vi "MAIN_CALLED_TESTASICS.vi"(8 "Error In":errorcluster, 11 "VISA resource name out":refnum<visa-resource-name>) -> (0 "Error Out":errorcluster)   [LabVIEW 2019]
uses:
  Type_defs/State_main.ctl
  LVPROJ_CONFIG_ESTACION/Type_defs/Coordenadas_estacion.ctl
  LVPROJ_CREAR BANDEJAS/Type_defs/Data_Bandeja.ctl
  Type_defs/INPUT TEST.ctl
  Type_defs/OUTPUTS_TEST.ctl
  LVPROJ_MOVIMIENTO_CABEZAL/LABVIEW_MOVIMIENTO/MOVIMIENTO CABEZAL/Typedefs/Comandos.ctl
  LVPROJ_MOVIMIENTO_CABEZAL/LABVIEW_MOVIMIENTO/MOVIMIENTO CABEZAL/Typedefs/Estados_arduino.ctl
  <vilib>/Utility/error.llb/Error Cluster From Error Code.vi
  <vilib>/ErrorRing/Error Ring.xnode
  SHARED VI'S/SHARED VI'S.lvlib
panel:
  out "trama datos enviada":string
  out "datos leídos por arduino":string
  in  "Tab Control":enum32{"PANEL USUARIO", "VER CONFIG ACTUAL"}(tab)
  in  "COMENZAR TEST":bool
  in  "EXIT":bool
  in  "DETENER TEST":bool
  in  "ENVIAR PARAMETROS DE TEST":bool
  in  "TEST ASICS INPUT":T1={"COORD. IN X"=0, "COORD IN Y"=0, "COORD OK X"=0, "COORD OK Y"=0, "COORD NOK X"=0, "COORD NOK Y"=0, "NºASICS A TESTEAR"=1, "SELECCIÓN DE TEST"=enum."TEST ASICS LST", "CUENTA ASICS"=0, "OPERADOR"="Javier Morales"}
  out "INDICADORES DE TEST":T2
  out "ESTADO FSM":T3
  in  "Path Out Reporte":path=path "C:/Trabajo_Robot/QC_LSTSUR"
  in  "Config file ASICS":path=path "C:/Trabajo_Robot/Test Asic Javi_2021/Origen Socket SERVO_PCB_BUENO_v5 (muchos asics)/CONFIG/configuracion_robot_CTAV2022A.test"
  in  "DIRECTORIO LOG FILE":path=path "C:/Trabajo_Robot/QC_LSTSUR/LOG/registro.txt"
  out "Configuracion Estación":T4={"Coordenadas_estacion"={"Coord.Bandeja entrada"={"Coord. X0 entrada"=0, "Coord. Y0 entrada "=0, "Altura Z entrada"=0}, "Coord.Bandeja OK"={"Coord. X0 OK"=0, "Coord. Y0 OK"=0, "Altura Z OK"=0}, "Coord.Bandeja entrada FAIL"={"Coord. X0 FAIL"=0, "Coord. Y0 FAIL"=0, "Altura Z FAIL"=0}, "Coord. Socket"={"Coord. X socket"=0, "Coord. Y socket"=0, "Altura Z socket"=0}}, "Nombre Bandeja"="", "Datos bandeja"={"Nº de columnas "=0, "Nº de filas "=0, "largo"=0, "ancho"=0, "nombre"="nombre", "Paso X (en mm)"=0.0, "Paso Y (en mm)"=0.0, "DISTANCIA SUELO A CHIP  "=0.0, "Nº de celdas totales"=0, "Distancia chips bandejas contiguas"=0.0}}
  out "read buffer":string
  out "read buffer 2":string
  out "datos enviados = datos leídos?":bool
  out "CONEXION CON ARDUINO":bool
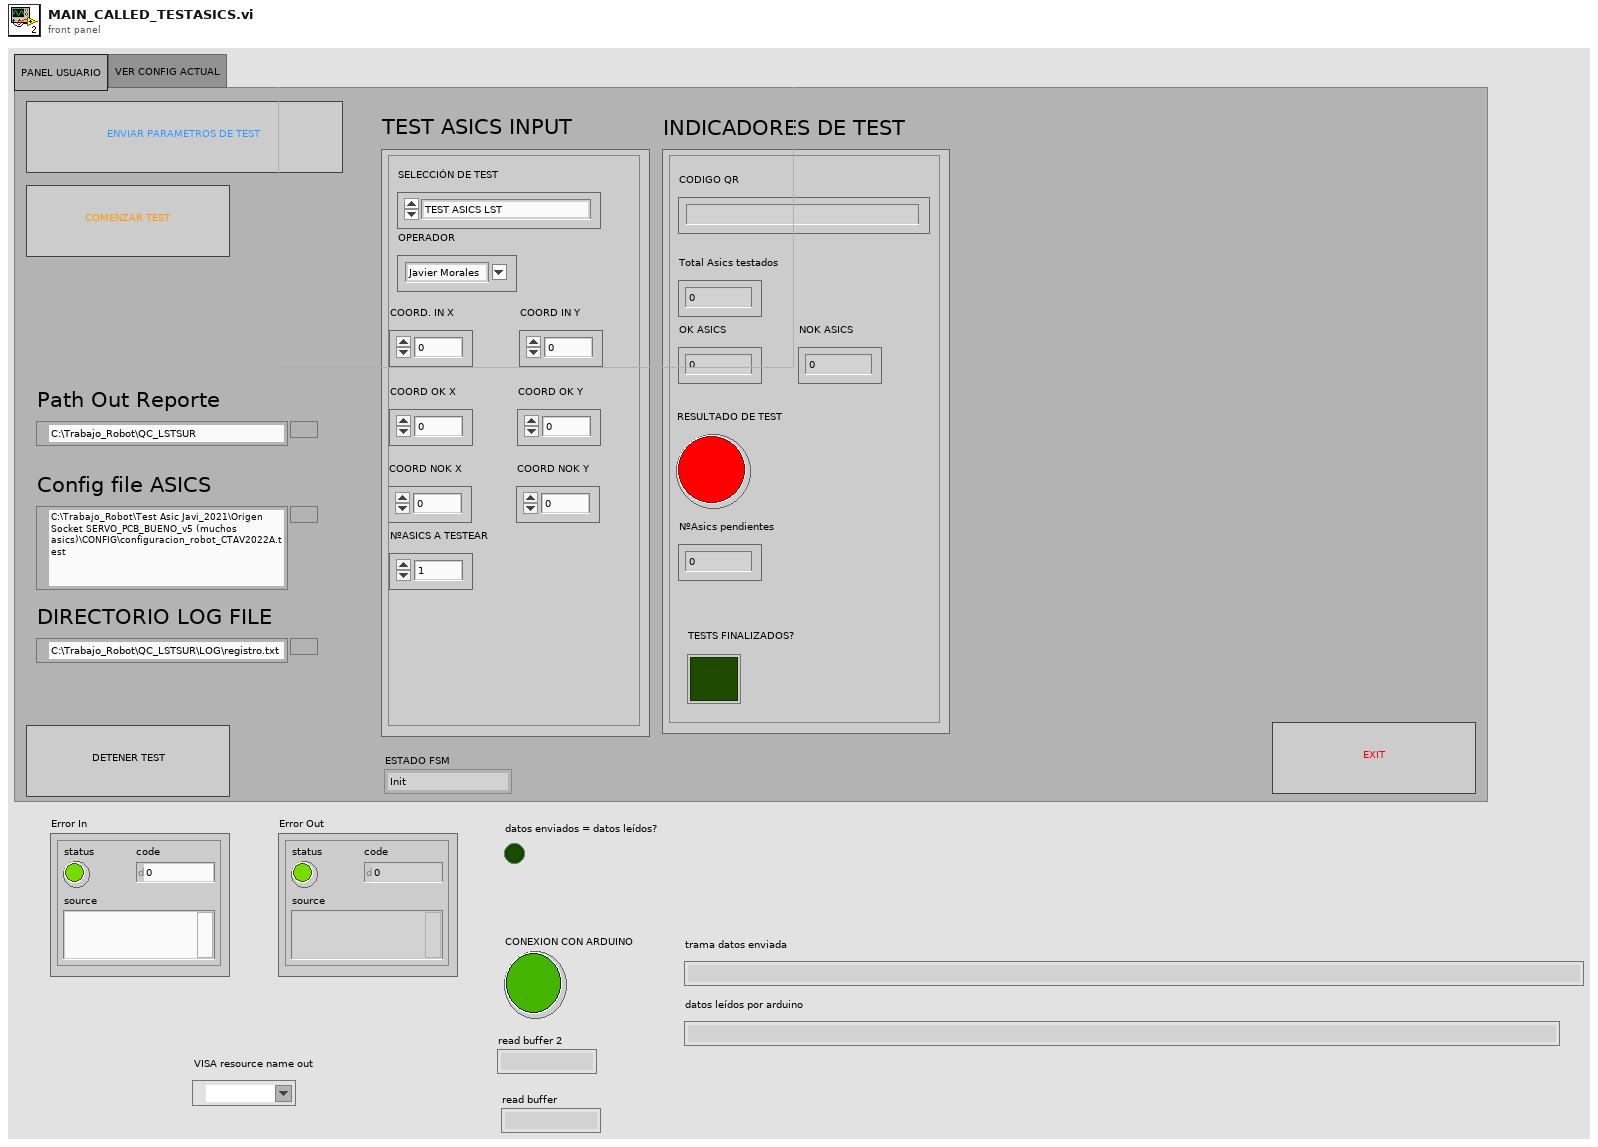
[diagram p1: front panel]
types:
  T1 = typedef "INPUT TEST.ctl" = cluster{"COORD. IN X":u16, "COORD IN Y":u16, "COORD OK X":u16, "COORD OK Y":u16, "COORD NOK X":u16, "COORD NOK Y":u16, "NºASICS A TESTEAR":u32, "SELECCIÓN DE TEST":enum16{"TEST ASICS LST"}, "CUENTA ASICS":u32, "OPERADOR":string}
  T2 = typedef "OUTPUTS_TEST.ctl" = cluster{"CODIGO QR":string, "OK ASICS":u32, "NOK ASICS":u32, "RESULTADO DE TEST":bool, "TESTS FINALIZADOS?":bool, "Total Asics testados":u32, "NºAsics pendientes":u32}
  T3 = typedef "State_main.ctl" = enum16{"Init", "Wait for Event", "Init refs", "Init com", "Config estacion", "Home", "Ping_Arduino", "Coge Asic", "Enviar_config_test", "Test_call", "Dejar Asic", "Leer QR", "Ejecutar Test", "Actualizar valores", "Enviar resultadoTest Arduino", "Final de test?", "Terminar", "Exit", "Error?"}
  T4 = typedef "Configuracion_estación.ctl" = cluster{"Coordenadas_estacion":T5, "Nombre Bandeja":string, "Datos bandeja":T6}
  T5 = typedef "Coordenadas_estacion.ctl" = cluster{"Coord.Bandeja entrada":cluster{"Coord. X0 entrada":u32, "Coord. Y0 entrada ":u32, "Altura Z entrada":u32}, "Coord.Bandeja OK":cluster{"Coord. X0 OK":u32, "Coord. Y0 OK":u32, "Altura Z OK":u32}, "Coord.Bandeja entrada FAIL":cluster{"Coord. X0 FAIL":u32, "Coord. Y0 FAIL":u32, "Altura Z FAIL":u32}, "Coord. Socket":cluster{"Coord. X socket":u32, "Coord. Y socket":u32, "Altura Z socket":u32}}
  T6 = typedef "Data_Bandeja.ctl" = cluster{"Nº de columnas ":u32, "Nº de filas ":u32, "largo":u32, "ancho":u32, "nombre":string, "Paso X (en mm)":dbl, "Paso Y (en mm)":dbl, "DISTANCIA SUELO A CHIP  ":dbl, "Nº de celdas totales":u16, "Distancia chips bandejas contiguas":dbl}
  T7 = typedef "Comandos.ctl" = enum16{"H", "FH", "FM", "FI", "FX", "FY", "FZ", "I", "OK"}
  T8 = typedef "Estados_arduino.ctl" = enum16{"2", "3", "4", "5", "6", "7", "9", "8"}
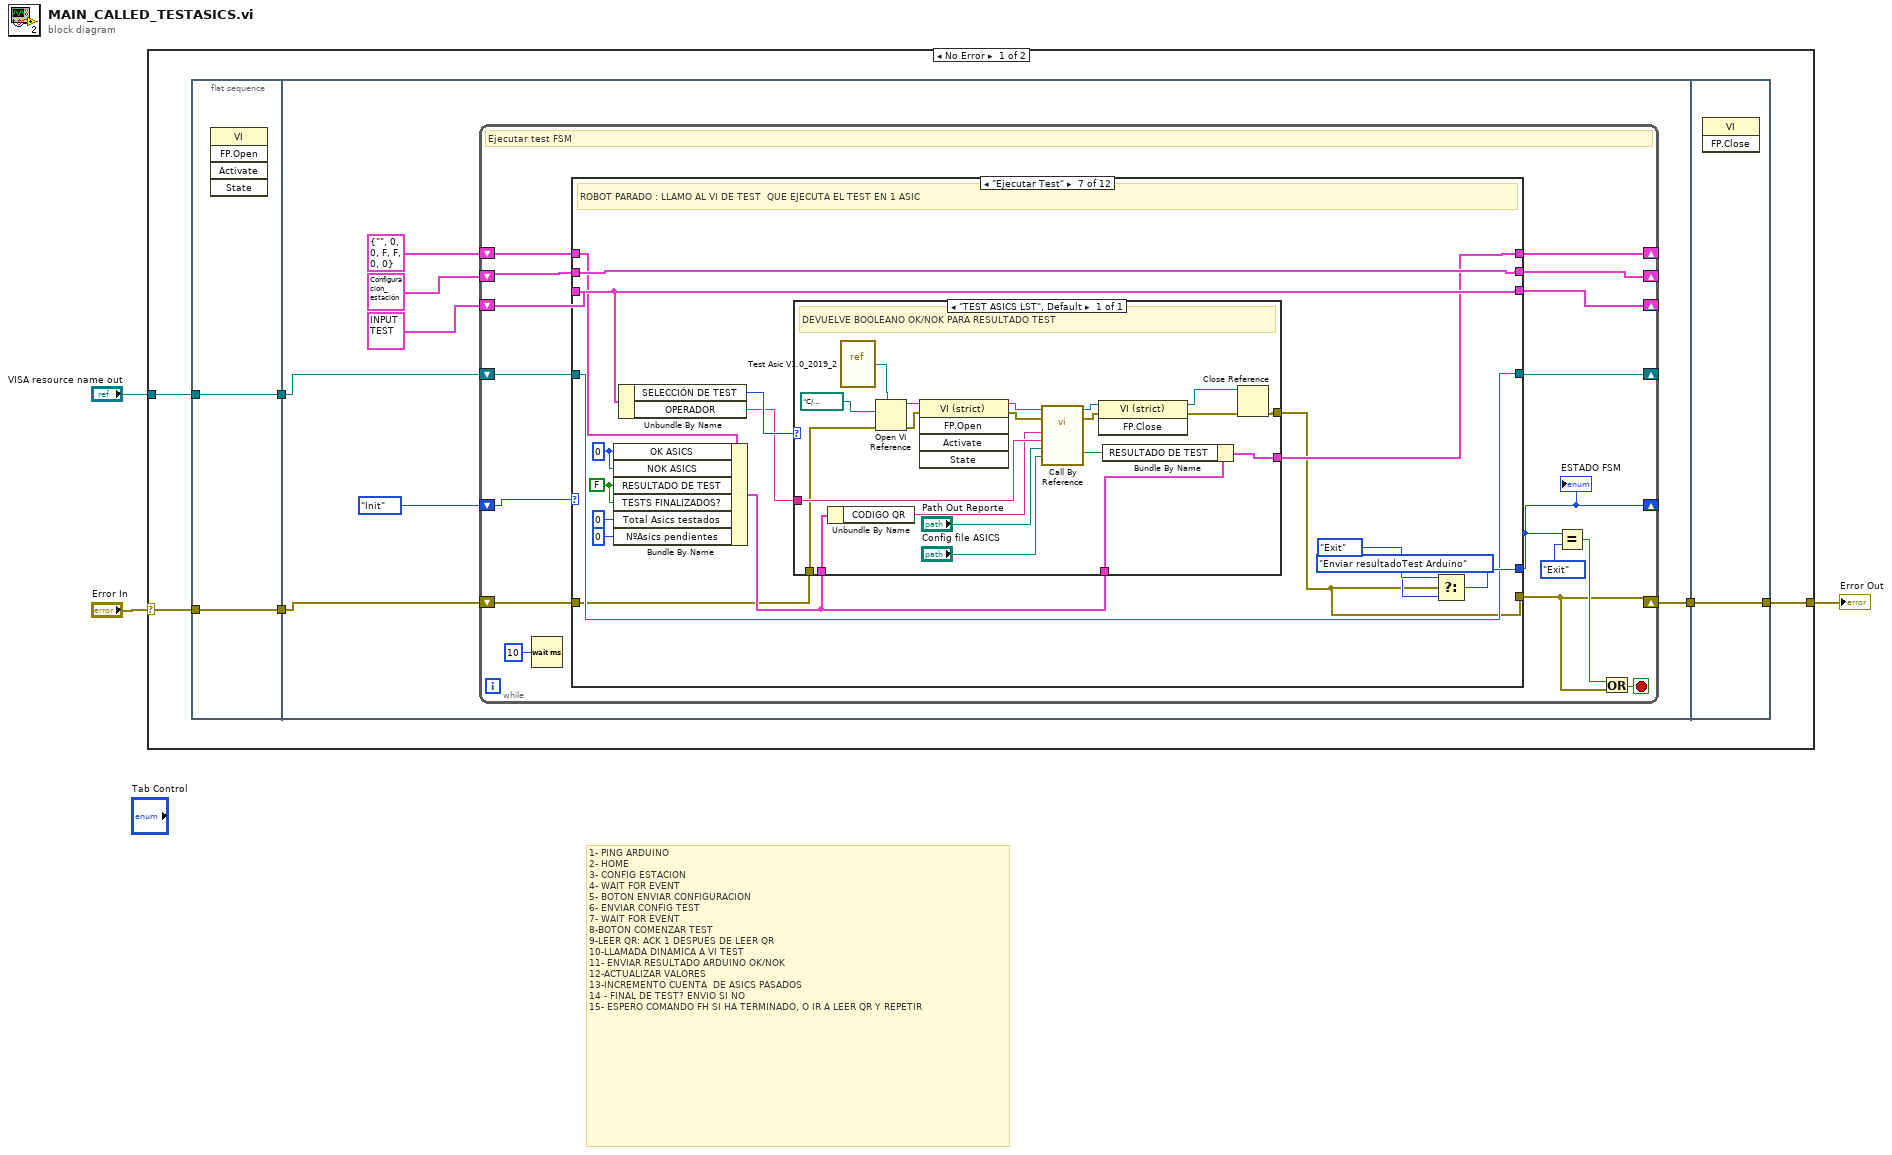
[diagram p0: block diagram]
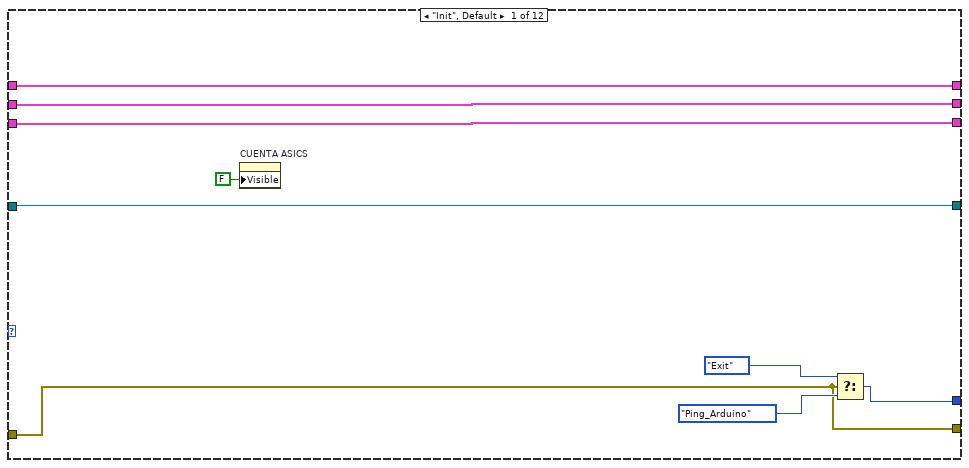
[diagram p2: hidden frame]
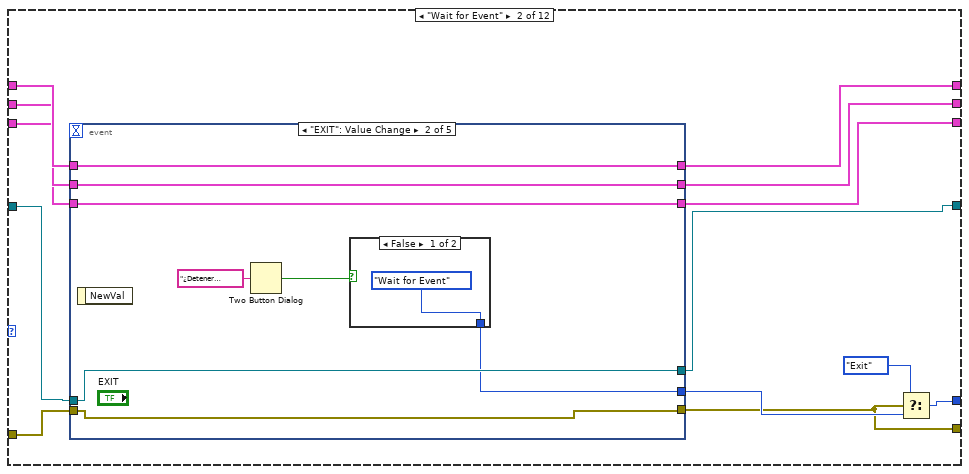
[diagram p3: hidden frame]
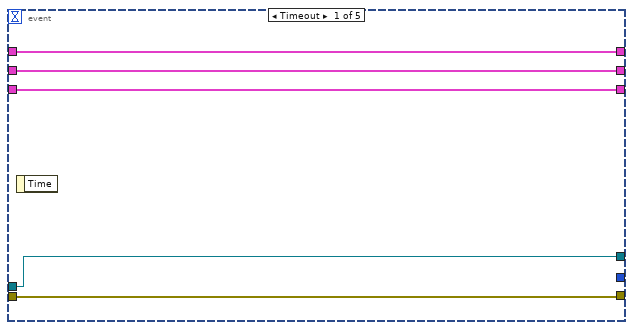
[diagram p4: hidden frame]
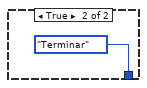
[diagram p5: hidden frame]
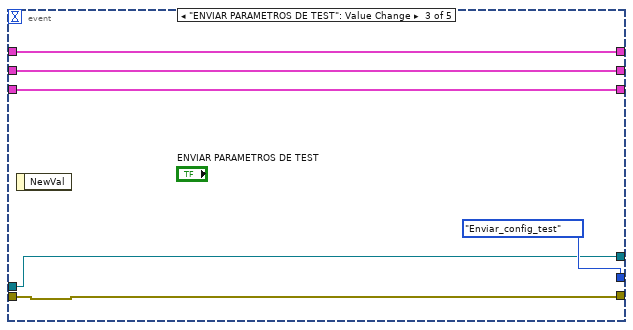
[diagram p6: hidden frame]
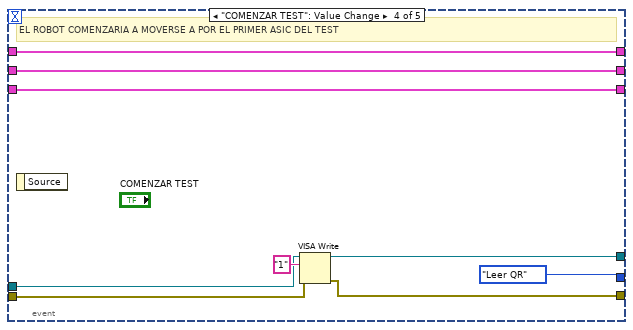
[diagram p7: hidden frame]
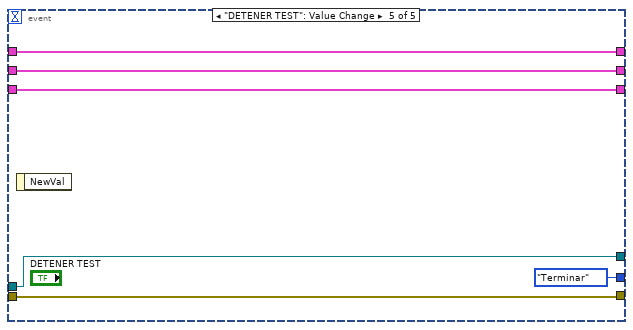
[diagram p8: hidden frame]
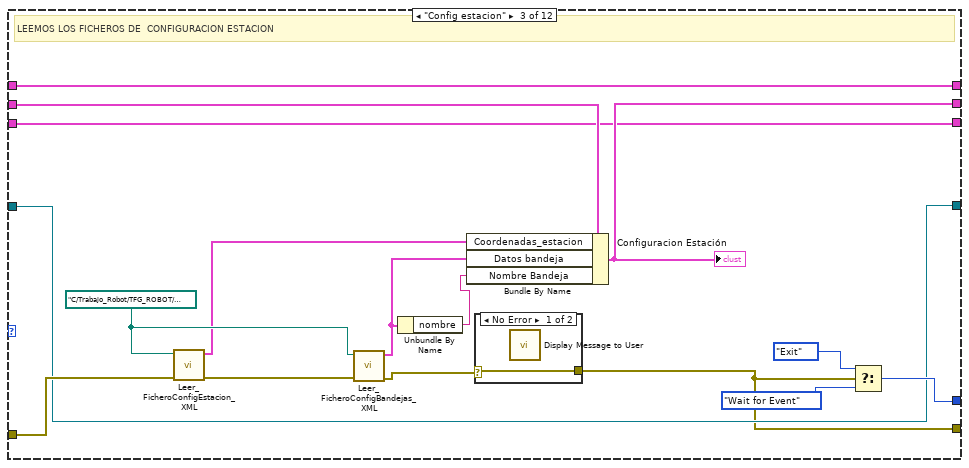
[diagram p9: hidden frame]
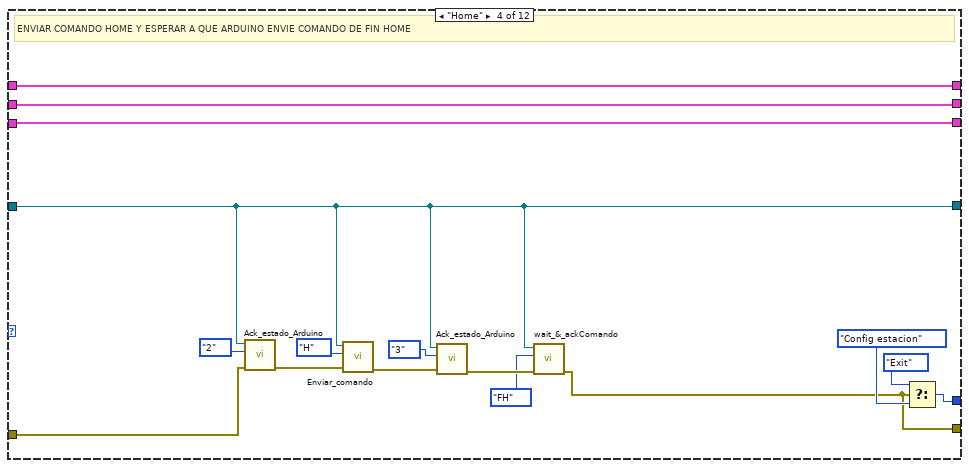
[diagram p11: hidden frame]
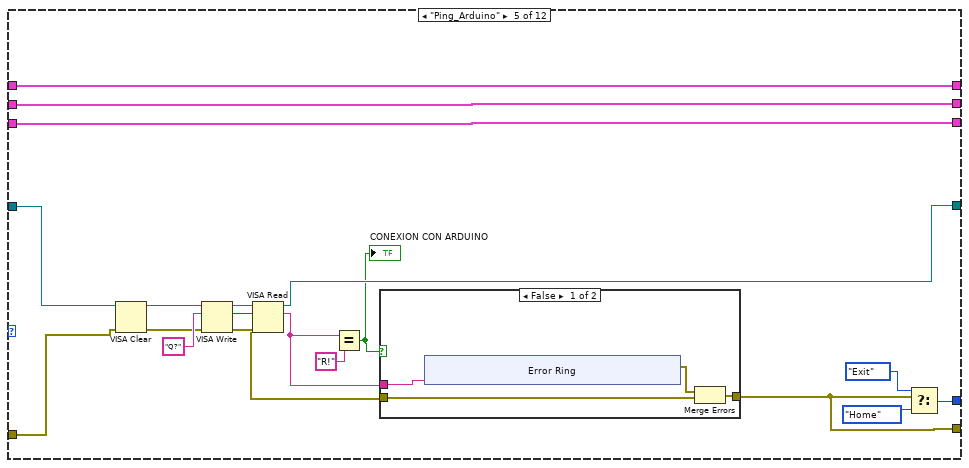
[diagram p12: hidden frame]
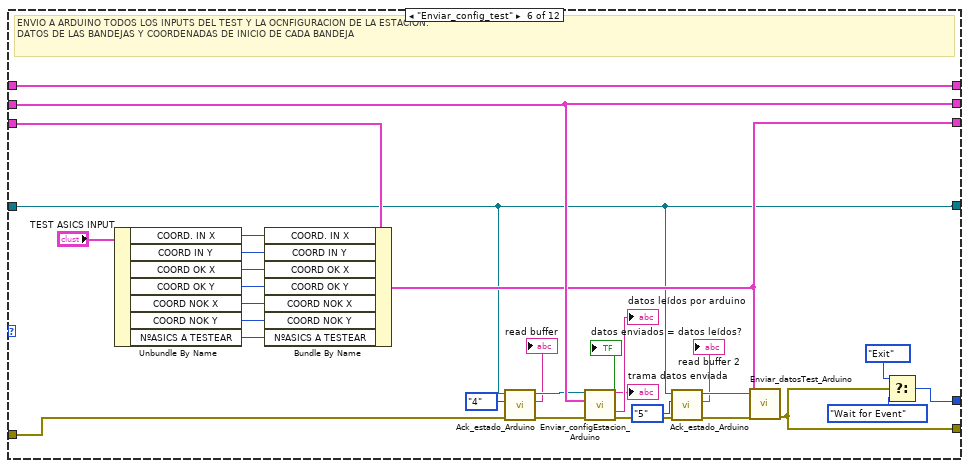
[diagram p14: hidden frame]
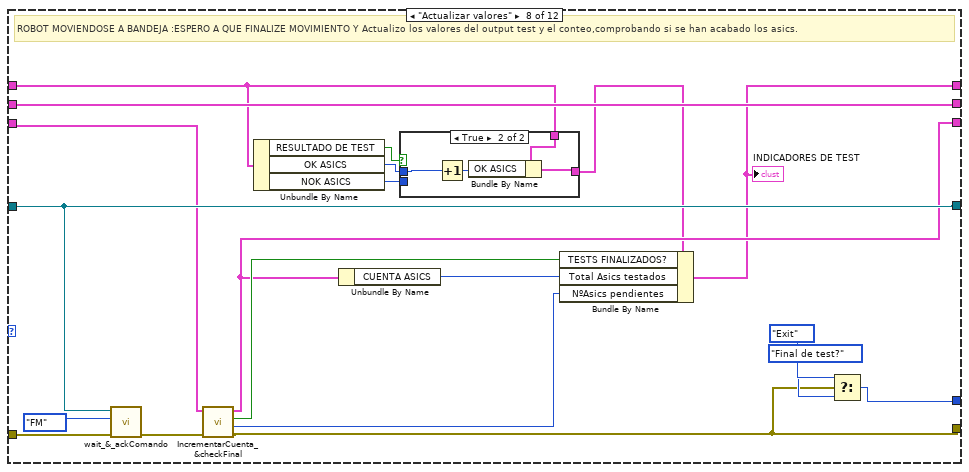
[diagram p15: hidden frame]
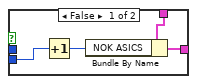
[diagram p16: hidden frame]
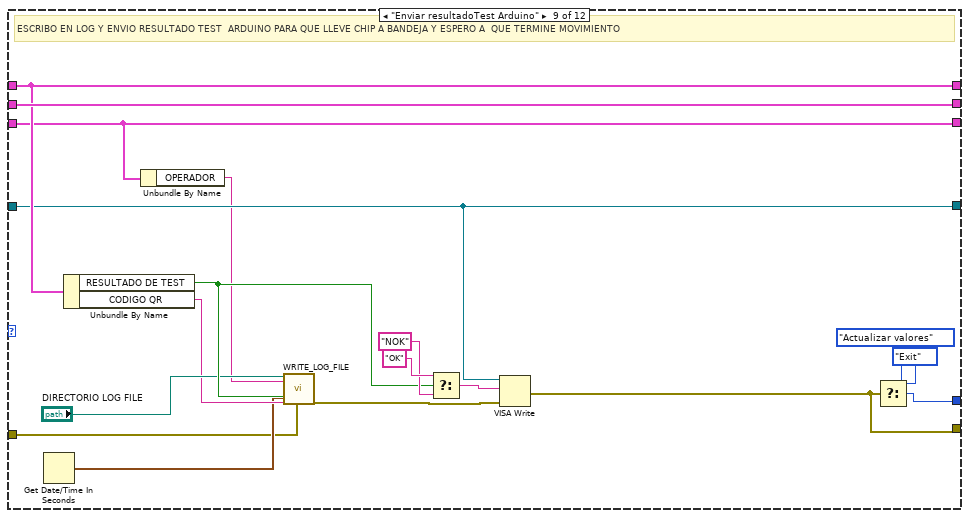
[diagram p17: hidden frame]
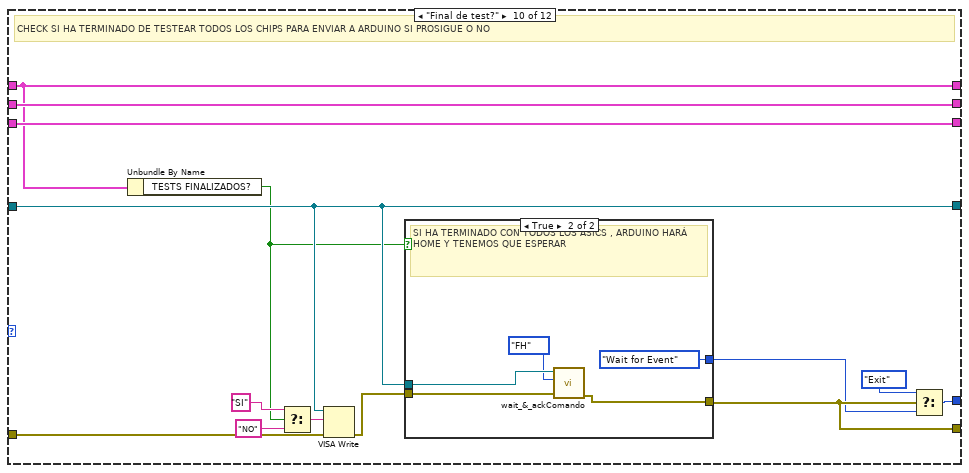
[diagram p18: hidden frame]
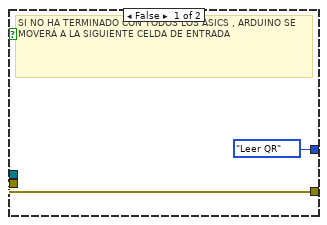
[diagram p19: hidden frame]
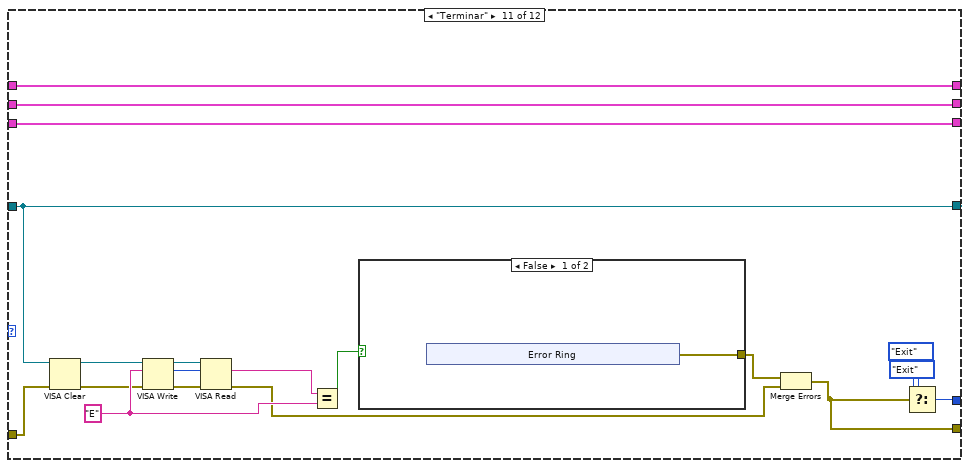
[diagram p20: hidden frame]
diagram:
  # "1- PING ARDUINO\n2- HOME\n3- CONFIG ESTACION\n4- WAIT FOR EVENT\n5- BOTON ENVIAR CONFIGURACION\n6- ENVIAR CONFIG TEST\n7- WAIT FOR EVENT\n8-BOTON COMENZAR TEST\n9-LEER QR: ACK 1 DESPUES DE LEER QR\n10-LLAMADA DINAMICA A VI TEST\n11- ENVIAR RESULTADO ARDUINO OK/NOK\n12-ACTUALIZAR VALORES\n13-INCREMENTO CUENTA  DE ASICS PASADOS\n14 - FINAL DE TEST? ENVIO SI NO\n15- ESPERO COMANDO FH SI HA TERMINADO, O IR A LEER QR Y REPETIR"
  n1 = case shown="No Error" "Error In" {
    selector: "Error In" -> [w9 w339]
    tunnel: "VISA resource name out" -> [w7 _]
    tunnel: [w4 w339] -> w1
    frame No Error {
      n2 = flat-sequence {
        tunnel: w9 -> [w11]
        tunnel: [w11] -> w8
        tunnel: w7 -> [w10]
        tunnel: [w10] -> w6
        tunnel: w8 -> [w14]
        tunnel: w6 -> [w13]
        tunnel: [w12] -> w5
        tunnel: w5 -> [w338]
        tunnel: [w338] -> w4
        frame #0 {
          n3 = invoke class="VI" method="FP.Open"() -> ()  [unwired: 5 in, 5 out]
        }
        frame #1 {
          n4 = while {
            shift-right: [w27] -> _
            shift-left: State_main."Init" ("States_main") -> [w34]
            shift-right: [w28] -> w12
            shift-left: w14 -> [w32]
            shift-right: [w20] -> _
            shift-left: T1 {"COORD. IN X"=0, "COORD IN Y"=0, "COORD OK X"=0, "COORD OK Y"=0, "COORD NOK X"=0, "COORD NOK Y"=0, "NºASICS A TESTEAR"=1, "SELECCIÓN DE TEST"=enum."TEST ASICS LST", "CUENTA ASICS"=0, "OPERADOR"="Javier Morales"} ("TEST ASICS INPUT") -> [w31]
            shift-right: [w22] -> _
            shift-left: T4 {"Coordenadas_estacion"={"Coord.Bandeja entrada"={"Coord. X0 entrada"=0, "Coord. Y0 entrada "=0, "Altura Z entrada"=0}, "Coord.Bandeja OK"={"Coord. X0 OK"=0, "Coord. Y0 OK"=0, "Altura Z OK"=0}, "Coord.Bandeja entrada FAIL"={"Coord. X0 FAIL"=0, "Coord. Y0 FAIL"=0, "Altura Z FAIL"=0}, "Coord. Socket"={"Coord. X socket"=0, "Coord. Y socket"=0, "Altura Z socket"=0}}, "Nombre Bandeja"="", "Datos bandeja"={"Nº de columnas "=0, "Nº de filas "=0, "largo"=0, "ancho"=0, "nombre"="nombre", "Paso X (en mm)"=0.0, "Paso Y (en mm)"=0.0, "DISTANCIA SUELO A CHIP  "=0.0, "Nº de celdas totales"=0, "Distancia chips bandejas contiguas"=0.0}} ("Configuracion Estación") -> [w26]
            shift-right: [w24] -> _
            shift-left: w13 -> [w25]
            shift-right: [w21] -> _
            shift-left: T2 {"CODIGO QR"="", "OK ASICS"=0, "NOK ASICS"=0, "RESULTADO DE TEST"=FALSE, "TESTS FINALIZADOS?"=FALSE, "Total Asics testados"=0, "NºAsics pendientes"=0} -> [w23]
            stop <- w30 stop-if-true
            # "Ejecutar test FSM"
            n5 = Wait (ms)(milliseconds to wait=u32 10) -> ()  [unwired: 1 out]
            n6 = case shown="\"Ejecutar Test\"" w34 {
              tunnel: w32 -> [w36 w47 w105 w114 w130 w171 w190 w240 w255 w278 w297 w328]
              tunnel: w31 -> [w38 w49 w95 w121 w141 w185 w200 w238 w258 w282 w307 w330]
              tunnel: [w41 w55 w106 w124 w144 w186 w203 w243 w269 w284 w306 w332] -> w27
              tunnel: [w36 w46 w93 w113 w133 w174 w189 w236 w262 w276 w293 w323] -> w28
              tunnel: w26 -> [w39 w51 w98 w122 w142 w175 w201 w242 w268 w283 w308 w331]
              tunnel: w25 -> [w37 w45 w99 w111 w128 w166 w199 w241 w263 w275 w296 w327]
              tunnel: [w37 w44 w99 w111 w132 w166 w199 w241 w263 w275 w296 w327] -> w24
              tunnel: w23 -> [w40 w53 w96 w123 w143 w176 w194 w229 w267 w272 w309 w326]
              tunnel: [w39 w50 w97 w122 w142 w175 w201 w242 w268 w283 w308 w331] -> w22
              tunnel: [w40 w52 w96 w123 w143 w176 w191 w231 w267 w272 w309 w325] -> w21
              tunnel: [w38 w48 w95 w121 w141 w173 w200 w234 w258 w282 w307 w330] -> w20
              frame "Init", Default {
                n7 = property on="CUENTA ASICS" class="DigNum (strict)"("Visible"=FALSE) -> ()  [unwired: 2 in, 2 out]
                n8 = Select(t=State_main."Exit" ("States_main"), s=w36, f=State_main."Ping_Arduino" ("States_main")) -> (s? t:f=w41:T3)
              }
              frame "Wait for Event" {
                n9 = event shown="[1] \"EXIT\": Value Change" {
                  selector: _ -> [_ _ _ _ _]
                  dyn-events: _ -> [_ _ _ _ _]
                  timeout: _ -> [_ _ _ _ _]
                  tunnel: [_ w62 State_main."Enviar_config_test" ("States_main") State_main."Leer QR" ("States_main") State_main."Terminar" ("States_main")] -> w54
                  tunnel: w53 -> [w61 w69 w76 w85 w92]
                  tunnel: [w61 w69 w76 w85 w92] -> w52
                  tunnel: w51 -> [w60 w68 w75 w84 w91]
                  tunnel: [w60 w68 w75 w84 w91] -> w50
                  tunnel: w49 -> [w59 w67 w74 w83 w90]
                  tunnel: [w59 w67 w74 w83 w90] -> w48
                  tunnel: w47 -> [w58 w66 w73 w79 w88]
                  tunnel: [w58 w66 w73 w78 w88] -> w46
                  tunnel: w45 -> [w57 w65 w72 w81 w87]
                  tunnel: [w57 w65 w72 w80 w87] -> w44
                  event Timeout {
                    n10 = event-data() -> ()  [unwired: 1 in, 1 out]
                  }
                  event "EXIT": Value Change {
                    n11 = event-data() -> ()  [unwired: 1 in, 1 out]
                    n12 = Two Button Dialog(message="¿Detener ejecución?") -> (T button?=w63:bool)  [unwired: 2 in]
                    n13 = case shown="False" w63 {
                      tunnel: [State_main."Wait for Event" ("States_main") State_main."Terminar" ("States_main")] -> w62
                      frame False {
                      }
                      frame True {
                      }
                    }
                  }
                  event "ENVIAR PARAMETROS DE TEST": Value Change {
                    n14 = event-data() -> ()  [unwired: 1 in, 1 out]
                  }
                  event "COMENZAR TEST": Value Change {
                    # "EL ROBOT COMENZARIA A MOVERSE A POR EL PRIMER ASIC DEL TEST"
                    n15 = event-data() -> ()  [unwired: 1 in, 1 out]
                    n16 = VISA Write(VISA resource name=w81, write buffer="1", error in (no error)=w79) -> (VISA resource name out=w80:refnum<visa-resource-name>, error out=w78:errorcluster)  [unwired: 1 out]
                  }
                  event "DETENER TEST": Value Change {
                    n17 = event-data() -> ()  [unwired: 1 in, 1 out]
                  }
                }
                n18 = Select(t=State_main."Exit" ("States_main"), s=w46, f=w54) -> (s? t:f=w55:T3)
              }
              frame "Config estacion" {
                w103 = path "C:/Trabajo_Robot/TFG_ROBOT/CONTROL_ROBOT/LABVIEW_ROBOT_MASTER" ("XML File Path")
                # "LEEMOS LOS FICHEROS DE  CONFIGURACION ESTACION"
                n19 = call "Leer_FicheroConfigEstacion_XML.vi"("error in (no error)"=w105, "XML File Path"=w103) -> ("error out"=w104:errorcluster, "Coordenadas_estacion"=w102:T5)  [unwired: 8 in]
                n20 = call "Leer_FicheroConfigBandejas_XML.vi"("error in (no error)"=w104, "XML File Path"=w103) -> ("error out"=w94:errorcluster, "Datos bandeja"=w101:T6)  [unwired: 8 in]
                n21 = Unbundle By Name(w101) -> ("nombre"=w100:string)
                n22 = Bundle By Name(cluster=w98, "Coordenadas_estacion"=w102, "Datos bandeja"=w101, "Nombre Bandeja"=w100) -> (w97:T4)
                "Configuracion Estación" <- w97
                n23 = case shown="No Error" w94 {
                  selector: w94 -> [w109 w110]
                  tunnel: [w109 w110] -> w93
                  frame No Error {
                    n24 = call "Display Message to User"() -> ()  [unwired: 10 in, 2 out]
                  }
                  frame Error {
                  }
                }
                n25 = Select(t=State_main."Exit" ("States_main"), s=w93, f=State_main."Wait for Event" ("States_main")) -> (s? t:f=w106:T3)
              }
              frame "Home" {
                # "ENVIAR COMANDO HOME Y ESPERAR A QUE ARDUINO ENVIE COMANDO DE FIN HOME"
                n26 = call "Ack_estado_Arduino.vi"("error in (no error)"=w114, "Enum"=Estados_arduino."2", "VISA resource name"=w111) -> ("error out"=w120:errorcluster)  [unwired: 6 in, 2 out]
                n27 = call "Enviar_comando.vi"("error in (no error)"=w120, "Enum"=Comandos."H", "VISA resource name"=w111) -> ("error out"=w115:errorcluster)  [unwired: 6 in, 2 out]
                n28 = call "Ack_estado_Arduino.vi"("error in (no error)"=w115, "Enum"=Estados_arduino."3", "VISA resource name"=w111) -> ("error out"=w116:errorcluster)  [unwired: 6 in, 2 out]
                n29 = call "wait_&_ackComando.vi"("error in (no error)"=w116, 10:Comandos."FH", "VISA Refnum in"=w111) -> ("error out"=w113:errorcluster)  [unwired: 7 in, 1 out]
                n30 = Select(t=State_main."Exit" ("States_main"), s=w113, f=State_main."Config estacion" ("States_main")) -> (s? t:f=w124:T3)
              }
              frame "Ping_Arduino" {
                n31 = VISA Clear(VISA resource name=w128, error in (no error)=w130) -> (VISA resource name out=w127:refnum<visa-resource-name>, error out=w129:errorcluster)
                n32 = VISA Write(VISA resource name=w127, write buffer="Q?", error in (no error)=w129) -> (VISA resource name out=w134:refnum<visa-resource-name>, return count=w139:u32, error out=w138:errorcluster)
                n33 = VISA Read(VISA resource name=w134, byte count=w139, error in (no error)=w138) -> (VISA resource name out=w132:refnum<visa-resource-name>, read buffer=w136:string, error out=w135:errorcluster)  [unwired: 1 out]
                n34 = Equal?(x=w136, y="R!") -> (x = y?=w131:bool)
                "CONEXION CON ARDUINO" <- w131
                n35 = case shown="False" w131 {
                  tunnel: w136 -> [w150 _]
                  tunnel: w135 -> [w148 w158]
                  tunnel: [w147 w158] -> w133
                  frame False {
                    n36 = xnode "Error Ring"("parameter 0"=w150) -> ("error out"=w149:errorcluster)
                    n37 = Merge Errors(w149, w148) -> (w147:errorcluster)
                  }
                  frame True {
                  }
                }
                n38 = Select(t=State_main."Exit" ("States_main"), s=w133, f=State_main."Home" ("States_main")) -> (s? t:f=w144:T3)
              }
              frame "Enviar_config_test" {
                # "ENVIO A ARDUINO TODOS LOS INPUTS DEL TEST Y LA OCNFIGURACION DE LA ESTACIÓN:\nDATOS DE LAS BANDEJAS Y COORDENADAS DE INICIO DE CADA BANDEJA"
                n39 = Unbundle By Name("TEST ASICS INPUT") -> ("COORD. IN X"=w183:u16, "COORD IN Y"=w182:u16, "COORD OK X"=w181:u16, "COORD OK Y"=w180:u16, "COORD NOK X"=w179:u16, "COORD NOK Y"=w178:u16, "NºASICS A TESTEAR"=w177:u32)
                n40 = Bundle By Name(cluster=w185, "COORD. IN X"=w183, "COORD IN Y"=w182, "COORD OK X"=w181, "COORD OK Y"=w180, "COORD NOK X"=w179, "COORD NOK Y"=w178, "NºASICS A TESTEAR"=w177) -> (w173:T1)
                n41 = call "Ack_estado_Arduino.vi"("error in (no error)"=w171, "Enum"=Estados_arduino."4", "VISA resource name"=w166) -> ("error out"=w170:errorcluster, "read buffer"=→"read buffer":string, "VISA resource name out"=w167:refnum<visa-resource-name>)  [unwired: 6 in]
                n42 = call "Enviar_configEstacion_Arduino.vi"("VISA resource name"=w167, "Configuracion Estación"=w175, "error in (no error)"=w170) -> ("trama datos enviada"=→"trama datos enviada":string, "datos enviados = datos leídos?"=→"datos enviados = datos leídos?":bool, "datos leídos"=→"datos leídos por arduino":string, "error IO"=w169:errorcluster)  [unwired: 9 in]
                n43 = call "Ack_estado_Arduino.vi"("error in (no error)"=w169, "Enum"=Estados_arduino."5", "VISA resource name"=w166) -> ("error out"=w168:errorcluster, "read buffer"=→"read buffer 2":string, "VISA resource name out"=w165:refnum<visa-resource-name>)  [unwired: 6 in]
                n44 = call "Enviar_datosTest_Arduino.vi"("error in (no error)"=w168, "TEST ASICS INPUT"=w173, "VISA resource name"=w165) -> ("error IO"=w174:errorcluster)  [unwired: 8 in]
                n45 = Select(t=State_main."Exit" ("States_main"), s=w174, f=State_main."Wait for Event" ("States_main")) -> (s? t:f=w186:T3)
              }
              frame "Ejecutar Test" {
                w195 = FALSE ("RESULTADO DE TEST")
                w198 = u32 0 ("OK ASICS")
                # "ROBOT PARADO : LLAMO AL VI DE TEST  QUE EJECUTA EL TEST EN 1 ASIC"
                n46 = Bundle By Name(cluster=w194, "OK ASICS"=w198, "NOK ASICS"=w198, "RESULTADO DE TEST"=w195, "TESTS FINALIZADOS?"=w195, "Total Asics testados"=u32 0, "NºAsics pendientes"=u32 0) -> (w192:T2)
                n47 = Unbundle By Name(w200) -> ("SELECCIÓN DE TEST"=w202:enum16{"TEST ASICS LST"}, "OPERADOR"=w193:string)
                n48 = case shown="\"TEST ASICS LST\", Default" w202 {
                  tunnel: w193 -> [w213]
                  tunnel: w192 -> [w212]
                  tunnel: w192 -> [w210]
                  tunnel: [w209] -> w191
                  tunnel: w190 -> [w208]
                  tunnel: [w207] -> w189
                  frame "TEST ASICS LST", Default {
                    # "DEVUELVE BOOLEANO OK/NOK PARA RESULTADO TEST"
                    n49 = Unbundle By Name(w212) -> ("CODIGO QR"=w211:string)
                    n50 = vi-ref "Test Asic V1.0_2019_2.vi"() -> (w224:refnum<vi>)
                    n51 = Open VI Reference(type specifier VI Refnum (for type only)=w224, vi path=path "C:/Trabajo_Robot/Test Asic Javi_2021/Test Asic V1.0_2019_2.vi", error in (no error)=w208) -> (vi reference=w223:refnum<vi>, error out=w221:errorcluster)  [unwired: 3 in]
                    n52 = invoke class="VI (strict)" method="FP.Open"(reference=w223, error in=w221) -> (reference out=w222:refnum<vi>, error out=w220:errorcluster)  [unwired: 3 in, 3 out]
                    n53 = call-by-ref "?"(reference=w222, error in=w220, "Config File"="Config file ASICS", "Path Out Report"="Path Out Reporte", "Operator's Name"=w213, "ASIC'S Number"=w211) -> (reference out=w219:refnum<vi>, error out=w218:errorcluster, "OK, Fault 2"=w206:bool)  [unwired: 1 in]
                    n54 = invoke class="VI (strict)" method="FP.Close"(reference=w219, error in=w218) -> (reference out=w217:refnum<vi>, error out=w216:errorcluster)  [unwired: 1 in, 1 out]
                    n55 = Bundle By Name(cluster=w210, "RESULTADO DE TEST"=w206) -> (w209:T2)
                    n56 = Close Reference(reference=w217, error in (no error)=w216) -> (error out=w207:errorcluster)
                  }
                }
                n57 = Select(t=State_main."Exit" ("States_main"), s=w189, f=State_main."Enviar resultadoTest Arduino" ("States_main")) -> (s? t:f=w203:T3)
              }
              frame "Actualizar valores" {
                # "ROBOT MOVIENDOSE A BANDEJA :ESPERO A QUE FINALIZE MOVIMIENTO Y Actualizo los valores del output test y el conteo,comprobando si se han acabado los asics."
                n58 = call "wait_&_ackComando.vi"("error in (no error)"=w240, 10:Comandos."FM", "VISA Refnum in"=w241) -> ("error out"=w237:errorcluster)  [unwired: 7 in, 1 out]
                n59 = call "IncrementarCuenta_&checkFinal.vi"("error in (no error)"=w237, "TEST ASICS INPUT in"=w238) -> ("error out"=w236:errorcluster, "Asics pendientes"=w232:u32, "FINAL ASICS??"=w235:bool, "TEST ASICS INPUT out"=w234:T1)  [unwired: 6 in]
                n60 = Unbundle By Name(w229) -> ("RESULTADO DE TEST"=w230:bool, "OK ASICS"=w228:u32, "NOK ASICS"=w227:u32)
                n61 = Unbundle By Name(w234) -> ("CUENTA ASICS"=w233:u32)
                n62 = case shown="True" w230 {
                  tunnel: w229 -> [w249 w253]
                  tunnel: w228 -> [_ w252]
                  tunnel: w227 -> [w248 _]
                  tunnel: [w246 w250] -> w226
                  frame False {
                    n63 = Increment(x=w248) -> (x+1=w247:u32)
                    n64 = Bundle By Name(cluster=w249, "NOK ASICS"=w247) -> (w246:T2)
                  }
                  frame True {
                    n65 = Increment(x=w252) -> (x+1=w251:u32)
                    n66 = Bundle By Name(cluster=w253, "OK ASICS"=w251) -> (w250:T2)
                  }
                }
                n67 = Bundle By Name(cluster=w226, "TESTS FINALIZADOS?"=w235, "Total Asics testados"=w233, "NºAsics pendientes"=w232) -> (w231:T2)
                "INDICADORES DE TEST" <- w231
                n68 = Select(t=State_main."Exit" ("States_main"), s=w236, f=State_main."Final de test?" ("States_main")) -> (s? t:f=w243:T3)
              }
              frame "Enviar resultadoTest Arduino" {
                # "ESCRIBO EN LOG Y ENVIO RESULTADO TEST  ARDUINO PARA QUE LLEVE CHIP A BANDEJA Y ESPERO A  QUE TERMINE MOVIMIENTO"
                n69 = Get Date/Time In Seconds() -> (seconds since 1Jan1904=w256:timestamp)
                n70 = Unbundle By Name(w267) -> ("RESULTADO DE TEST"=w261:bool, "CODIGO QR"=w259:string)
                n71 = Unbundle By Name(w258) -> ("OPERADOR"=w257:string)
                n72 = call "WRITE_LOG_FILE.vi"("file path (use dialog)"="DIRECTORIO LOG FILE", "OPERADOR"=w257, "Resultado test"=w261, "ASIC QR CODE"=w259, "HORA COMIENZO"=w256, "error in"=w255) -> ("error out"=w254:errorcluster)  [unwired: 13 in]
                n73 = Select(t="OK", s=w261, f="NOK") -> (s? t:f=w264:string)
                n74 = VISA Write(VISA resource name=w263, write buffer=w264, error in (no error)=w254) -> (error out=w262:errorcluster)  [unwired: 2 out]
                n75 = Select(t=State_main."Exit" ("States_main"), s=w262, f=State_main."Actualizar valores" ("States_main")) -> (s? t:f=w269:T3)
              }
              frame "Final de test?" {
                # "CHECK SI HA TERMINADO DE TESTEAR TODOS LOS CHIPS PARA ENVIAR A ARDUINO SI PROSIGUE O NO"
                n76 = Unbundle By Name(w272) -> ("TESTS FINALIZADOS?"=w273:bool)
                n77 = Select(t="SI", s=w273, f="NO") -> (s? t:f=w279:string)
                n78 = VISA Write(VISA resource name=w275, write buffer=w279, error in (no error)=w278) -> (error out=w277:errorcluster)  [unwired: 2 out]
                n79 = case shown="True" w273 {
                  tunnel: w277 -> [w287 w290]
                  tunnel: [w287 w288] -> w276
                  tunnel: w275 -> [_ w291]
                  tunnel: [State_main."Leer QR" ("States_main") State_main."Wait for Event" ("States_main")] -> w274
                  frame False {
                    # "SI NO HA TERMINADO CON TODOS LOS ASICS , ARDUINO SE MOVERÁ A LA SIGUIENTE CELDA DE ENTRADA"
                  }
                  frame True {
                    # "SI HA TERMINADO CON TODOS LOS ASICS , ARDUINO HARÁ HOME Y TENEMOS QUE ESPERAR"
                    n80 = call "wait_&_ackComando.vi"("error in (no error)"=w290, 10:Comandos."FH", "VISA Refnum in"=w291) -> ("error out"=w288:errorcluster)  [unwired: 7 in, 1 out]
                  }
                }
                n81 = Select(t=State_main."Exit" ("States_main"), s=w276, f=w274) -> (s? t:f=w284:T3)
              }
              frame "Terminar" {
                w303 = "E" ("write buffer")
                n82 = VISA Clear(VISA resource name=w296, error in (no error)=w297) -> (VISA resource name out=w295:refnum<visa-resource-name>, error out=w301:errorcluster)
                n83 = VISA Write(VISA resource name=w295, write buffer=w303, error in (no error)=w301) -> (VISA resource name out=w294:refnum<visa-resource-name>, return count=w305:u32, error out=w302:errorcluster)
                n84 = VISA Read(VISA resource name=w294, byte count=w305, error in (no error)=w302) -> (read buffer=w304:string, error out=w298:errorcluster)  [unwired: 2 out]
                n85 = Equal?(x=w304, y=w303) -> (x = y?=w300:bool)
                n86 = case shown="False" w300 {
                  tunnel: [w312 _] -> w299
                  frame False {
                    n87 = xnode "Error Ring"() -> ("error out"=w312:errorcluster)
                  }
                  frame True {
                    n88 = call "Time Delay"() -> ()  [unwired: 11 in, 1 out]
                  }
                }
                n89 = Merge Errors(w299, w298) -> (w293:errorcluster)
                n90 = Select(t=State_main."Exit" ("States_main"), s=w293, f=State_main."Exit" ("States_main")) -> (s? t:f=w306:T3)
              }
              frame "Leer QR" {
                # "ROBOT MOVIENDOSE : ESPERO A QUE ARDUINO POSICIONE EL ASIC Y ME ENVIE EL FLAG = 1 PARA LEER EL QR"
                n91 = call "wait_&ackChar.vi"("error in (no error)"=w328, "caracter"="1", "VISA Refnum in"=w327) -> ("error out"=w321:errorcluster)  [unwired: 7 in, 1 out]
                n92 = for {
                  N: 3 -> [_]
                  tunnel: w321 -> [w336]
                  tunnel: [w337] -> w320
                  tunnel: [w336] -> w319
                  tunnel: [w335] -> w318
                  stop <- w335 stop-if-true
                  n93 = call "CapturaImagenyQR_subVI_pruebas.vi"() -> ("código leído?"=w335:bool, "Datos_QR"=w337:string)  [unwired: 9 in, 1 out]
                }
                n94 = Bundle By Name(cluster=w326, "CODIGO QR"=w320) -> (w325:T2)
                n95 = call "QR_error_generator.vi"("Error In"=w319, "CODIGO QR LEÍDO?"=w318) -> ("Error Out"=w323:errorcluster)  [unwired: 9 in]
                n96 = Unbundle By Name(w325) -> ("CODIGO QR"=w324:string)
                n97 = property on="CODIGO QR" class="Str"("Value"=w324) -> ()  [unwired: 2 in, 2 out]
                n98 = Select(t=State_main."Exit" ("States_main"), s=w323, f=State_main."Ejecutar Test" ("States_main")) -> (s? t:f=w332:T3)
              }
            }
            "ESTADO FSM" <- w27
            n99 = Equal?(x=w27, y=State_main."Exit") -> (x = y?=w33:bool)
            n100 = Or(x=w33, y=w28) -> (x .or. y?=w30:bool)
          }
        }
        frame #2 {
          n101 = invoke class="VI" method="FP.Close"() -> ()  [unwired: 3 in, 3 out]
        }
      }
    }
    frame Error {
    }
  }
  "Error Out" <- w1
